vi "niFpgaScaledWinOutsideSCTL.vi"(0 "real data in":fxp<+/-,24,1>, 1 "reset":bool, 5 "imaginary data in":fxp<+/-,24,1>) -> (3 "data index":u16, 4 "real data out":fxp<+/-,24,-1>, 6 "imaginary data out":fxp<+/-,24,-1>)   [LabVIEW 2017]
uses:
  <vilib>/Platform/TimedLoop/XDataNode/timing_clust.ctl
  <vilib>/Platform/TimedLoop/XDataNode/nitl_modes.ctl
  <vilib>/Platform/TimedLoop/XDataNode/wakeup.ctl
  <vilib>/Platform/TimedLoop/XDataNode/XDataNode.xnode
  <vilib>/rvi/FXPMathLib/basic elements/FxpDiscreteDelay/XNode/nifxpmath_DiscreteDelay.xnode
  <vilib>/rvi/FXPMathLib/FxpMul/XNode/nifxpmath_Multiplier.xnode
  <vilib>/Platform/TimedLoop/XDataNode/XDNodeRunTimeDep.lvlib
  <vilib>/rvi/FXPMathLib/sim/FxpSim.dll
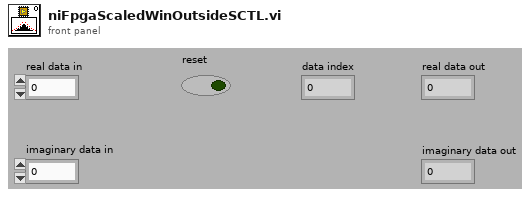
[diagram p1: front panel]
types:
  T1 = typedef "XDNodeRunTimeDep.lvlib/timing_clust.ctl" = cluster{"Expected End [f-1]":u64, "Actual End [f-1]":u64, "Finished Late? [f-1]":bool, "Expected End [i-1]":u64, "Actual End [i-1]":u64, "Finished Late? [i-1]":bool, "Expected Start [i]":u64, "Actual Start [i]":u64, "Expected Start [f]":u64, "Actual Start [f]":u64, "Source Name":string, "Structure Name":string, "Period":i64, "Deadline":i64, "Offset":i64, "Start":i64, "Priority":i32, "Timeout":i32, "Mode":T2, "Wakeup Reason":T3, "Error":errorcluster, "Source Type":string, "Secondary Source Type":string, "Global End Time":u64, "Global Start Time":u64, "Frame Duration":u64, "Iteration Duration":u64, "Assigned CPU":i32, "I/O Scan Engine Mode":u32}
  T2 = typedef "XDNodeRunTimeDep.lvlib/nitl_modes.ctl" = enum32{"No Change", "Process missed periods, maintain original phase", "Discard missed periods, maintain original phase", "Process missed periods, ignore original phase", "Discard missed periods, ignore original phase"}
  T3 = typedef "XDNodeRunTimeDep.lvlib/wakeup.ctl" = enum32{"Normal", "Aborted", "Asynchronous wakeup", "Timing source error", "Timed loop error", "Timeout"}
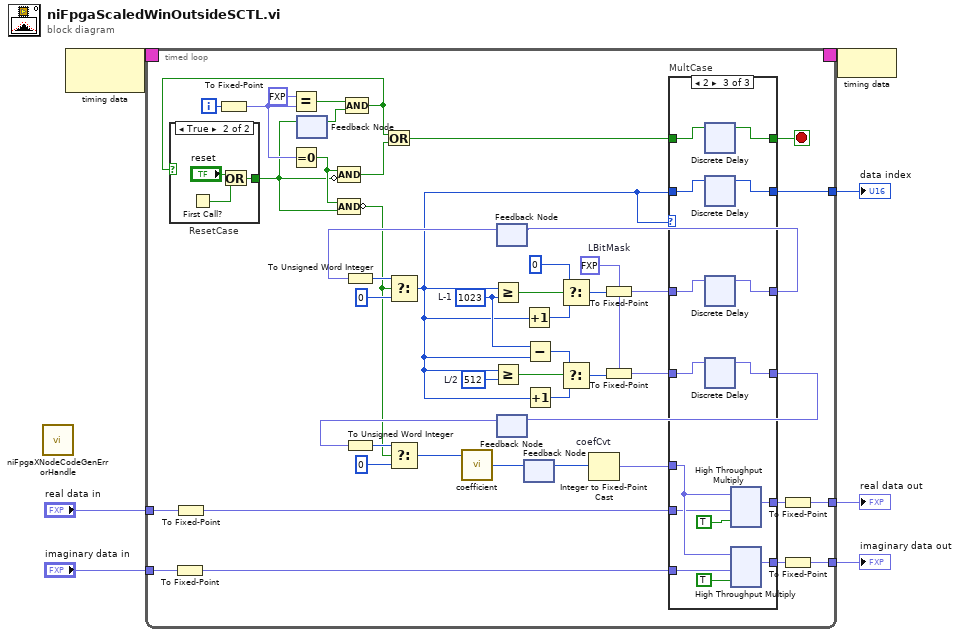
[diagram p0: block diagram]
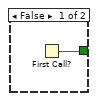
[diagram p2: hidden frame]
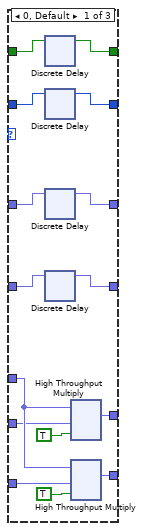
[diagram p3: hidden frame]
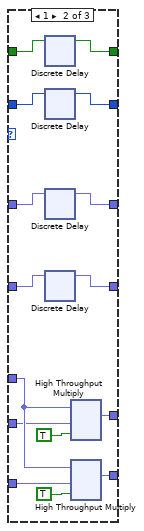
[diagram p4: hidden frame]
diagram:
  n1 = call <vilib>:"niFpgaXNodeCodeGenErrorHandle.vi"() -> ()  [unwired: 1 in]
  n2 = node-c288() -> (w2:T1)  [unwired: 1 out]
  n3 = timed-loop "MainLoop" {
    tunnel: "real data in" -> [w34]
    tunnel: [w33] -> w6
    tunnel: "imaginary data in" -> [w11]
    tunnel: [w32] -> w3
    tunnel: [w30] -> w4
    timing: w2 -> [_]
    timing-out: [_] -> w1
    i -> [w50]
    stop <- w15 stop-if-true
    w42 = fxp<+,11,11> 0.0  # LBitMask
    w46 = u16 1023  # L-1
    w49 = u16 512  # L/2
    n4 = To Fixed-Point(number=w11) -> (fixed-point=w10:fxp<+/-,24,1>)  [unwired: 1 in]
    n5 = To Fixed-Point(number=w34) -> (fixed-point=w12:fxp<+/-,24,1>)  [unwired: 1 in]
    n6 = To Fixed-Point(number=w50) -> (fixed-point=w20:fxp<+,3,3>)  [unwired: 1 out]
    n7 = Equal?(x=fxp<+,3,3> 1.0, y=w20) -> (x = y?=w22:bool)
    n8 = Equal To 0?(x=w20) -> (x = 0?=w25:bool)
    n9 = feedback #1() -> (w23:bool)  [unwired: 1 out]
    n10 = Compound Arithmetic op=AND(w22, w23) -> (w13:bool)
    n11 = case "ResetCase" shown="True" w13 {
      tunnel: [w55 w56] -> w19
      frame False {
        n12 = First Call?() -> (First Call?: T/F=w55:bool)
      }
      frame True {
        n13 = First Call?() -> (First Call?: T/F=w58:bool)
        n14 = Or(x="reset", y=w58) -> (x .or. y?=w56:bool)
      }
    }
    n15 = feedback-in #1(w19) -> ()
    n16 = Compound Arithmetic op=AND(w25, invert w19) -> (w24:bool)
    n17 = Compound Arithmetic op=AND(w25, w19) -> (invert w18:bool)
    n18 = Or(x=w13, y=w24) -> (x .or. y?=w16:bool)
    n19 = feedback #2() -> (w36:fxp<+,11,11>)  [unwired: 1 in]
    n20 = To Unsigned Word Integer(number=w36) -> (unsigned 16bit integer=w38:u16)
    n21 = Select(t=w38, s=w18, f=u16 0) -> (s? t:f=w14:u16)
    n22 = Greater Or Equal?(x=w14, y=w46) -> (x >= y?=w51:bool)
    n23 = Greater Or Equal?(x=w14, y=w49) -> (x >= y?=w52:bool)
    n24 = feedback #3() -> (w35:fxp<+,11,11>)  [unwired: 1 in]
    n25 = To Unsigned Word Integer(number=w35) -> (unsigned 16bit integer=w41:u16)
    n26 = Select(t=w41, s=w18, f=u16 0) -> (s? t:f=w43:u16)
    n27 = call "coefficient"("address"=w43) -> ("data out"=w37:i32)  [unwired: 8 in]
    n28 = Increment(x=w14) -> (x+1=w53:u16)
    n29 = feedback-in #4(w37) -> ()
    n30 = feedback #4() -> (w9:i32)  [unwired: 1 out]
    n31 = Subtract(x=w46, y=w14) -> (x-y=w48:u16)
    n32 = Increment(x=w14) -> (x+1=w47:u16)
    n33 = Select(t=u16 0, s=w51, f=w53) -> (s? t:f=w45:u16)
    n34 = Select(t=w48, s=w52, f=w47) -> (s? t:f=w44:u16)
    n35 = Integer to Fixed-Point Cast "coefCvt"(integer=w9) -> (fixed-point=w8:fxp<+/-,32,32>)  [unwired: 1 in]
    n36 = To Fixed-Point(fixed-point type=w42, number=w45) -> (fixed-point=w29:fxp<+,11,11>)
    n37 = To Fixed-Point(fixed-point type=w42, number=w44) -> (fixed-point=w27:fxp<+,11,11>)
    n38 = case "MultCase" shown="2" w14 {
      tunnel: [w73 w88 w103] -> w17
      tunnel: [w72 w87 w102] -> w31
      tunnel: w8 -> [w71 w86 w101]
      tunnel: w12 -> [w67 w82 w97]
      tunnel: w10 -> [w68 w83 w98]
      tunnel: w14 -> [w66 w81 w96]
      tunnel: [w65 w80 w95] -> w30
      tunnel: w29 -> [w64 w79 w94]
      tunnel: [w63 w78 w93] -> w28
      tunnel: w27 -> [w62 w77 w92]
      tunnel: [w61 w76 w91] -> w26
      tunnel: w16 -> [w60 w75 w90]
      tunnel: [w59 w74 w89] -> w15
      frame 0, Default {
        n39 = xnode "Discrete Delay"("D"=w60) -> ("Q"=w59:bool)
        n40 = xnode "Discrete Delay"("D"=w66) -> ("Q"=w65:u16)
        n41 = xnode "Discrete Delay"("D"=w64) -> ("Q"=w63:fxp<+,11,11>)
        n42 = xnode "Discrete Delay"("D"=w62) -> ("Q"=w61:fxp<+,11,11>)
        n43 = xnode "High Throughput Multiply"("x"=w71, "y"=w67, "input valid"=TRUE) -> ("x*y"=w73:fxp<+/-,56,33>)  [unwired: 1 in, 2 out]
        n44 = xnode "High Throughput Multiply"("x"=w71, "y"=w68, "input valid"=TRUE) -> ("x*y"=w72:fxp<+/-,56,33>)  [unwired: 1 in, 2 out]
      }
      frame 1 {
        n45 = xnode "Discrete Delay"("D"=w75) -> ("Q"=w74:bool)
        n46 = xnode "Discrete Delay"("D"=w81) -> ("Q"=w80:u16)
        n47 = xnode "Discrete Delay"("D"=w79) -> ("Q"=w78:fxp<+,11,11>)
        n48 = xnode "Discrete Delay"("D"=w77) -> ("Q"=w76:fxp<+,11,11>)
        n49 = xnode "High Throughput Multiply"("x"=w86, "y"=w82, "input valid"=TRUE) -> ("x*y"=w88:fxp<+/-,56,33>)  [unwired: 1 in, 2 out]
        n50 = xnode "High Throughput Multiply"("x"=w86, "y"=w83, "input valid"=TRUE) -> ("x*y"=w87:fxp<+/-,56,33>)  [unwired: 1 in, 2 out]
      }
      frame 2 {
        n51 = xnode "Discrete Delay"("D"=w90) -> ("Q"=w89:bool)
        n52 = xnode "Discrete Delay"("D"=w96) -> ("Q"=w95:u16)
        n53 = xnode "Discrete Delay"("D"=w94) -> ("Q"=w93:fxp<+,11,11>)
        n54 = xnode "Discrete Delay"("D"=w92) -> ("Q"=w91:fxp<+,11,11>)
        n55 = xnode "High Throughput Multiply"("x"=w101, "y"=w97, "input valid"=TRUE) -> ("x*y"=w103:fxp<+/-,56,33>)  [unwired: 1 in, 2 out]
        n56 = xnode "High Throughput Multiply"("x"=w101, "y"=w98, "input valid"=TRUE) -> ("x*y"=w102:fxp<+/-,56,33>)  [unwired: 1 in, 2 out]
      }
    }
    n57 = feedback-in #2(w28) -> ()
    n58 = feedback-in #3(w26) -> ()
    n59 = To Fixed-Point ("MultCast")(number=w17) -> (fixed-point=w33:fxp<+/-,24,-1>)  [unwired: 1 out]
    n60 = To Fixed-Point ("MultCast")(number=w31) -> (fixed-point=w32:fxp<+/-,24,-1>)  [unwired: 1 out]
  }
  "data index" <- w4
  "real data out" <- w6
  "imaginary data out" <- w3
  n61 = node-c288(w1) -> ()
